vi "Execute.vi"(8 "error in (no error)":errorcluster, 11 "Data Source in":refnum<class "Component.lvclass">) -> (0 "error out":errorcluster, 2 "Data":dbl[](array[numeric]), 3 "Data Source out":refnum<class "Component.lvclass">)   [LabVIEW 2021, in "Component.lvclass"]
uses:
  Component.lvclass
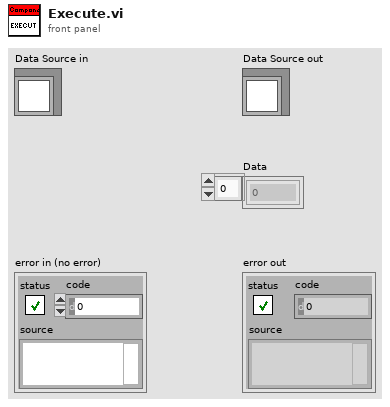
[diagram p1: front panel]
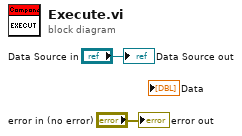
[diagram p0: block diagram]
diagram:
  "error out" <- "error in (no error)"
  "Data Source out" <- "Data Source in"
